vi "1-Coin Toss.vi"() -> ()   [LabVIEW 2014]
panel:
  out "RNG Value":dbl
  out "Coin Toss!!!":string
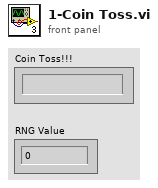
[diagram p1: front panel]
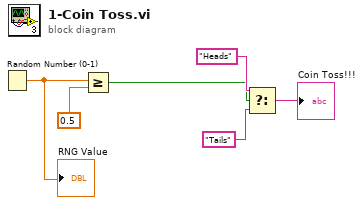
[diagram p0: block diagram]
diagram:
  n1 = Random Number (0-1)() -> (number: 0 to 1=w1:dbl)
  "RNG Value" <- w1
  n2 = Greater Or Equal?(x=w1, y=0.5) -> (x >= y?=w3:bool)
  n3 = Select(t="Heads", s=w3, f="Tails") -> (s? t:f=→"Coin Toss!!!":string)
